vi "DAQ6363_SetCORestLevel.vi"(8 "error in (no error)":errorcluster caption="entrée d'erreur (pas d'erreur)", 10 "CO.Impulsion.ÉtatRepos":i32(ring)=10192 items=["Haut"=10192, "Bas"=10214], 11 "TaskIn":refnum<k21>) -> (0 "error out":errorcluster caption="sortie d'erreur", 3 "TaskOut":refnum<k21>)   [LabVIEW 2019]
uses:
  <resource>/objmgr/daqmx.rc
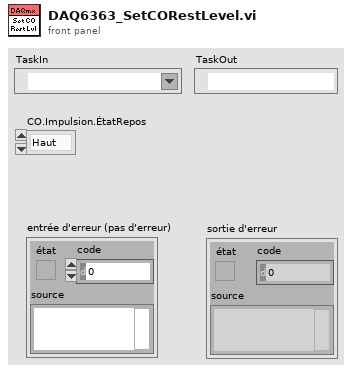
[diagram p1: front panel]
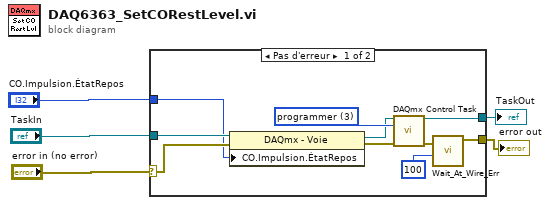
[diagram p0: block diagram]
diagram:
  n1 = case shown="Pas d'erreur" "error in (no error)" {
    selector: "error in (no error)" -> [w7 w16]
    tunnel: [w10 w16] -> w2
    tunnel: "TaskIn" -> [w9 w17]
    tunnel: [w8 w17] -> w3
    tunnel: "CO.Impulsion.ÉtatRepos" -> [w6 _]
    frame No Error {
      w15 = 3 items=["vérifier"=2, "réserver"=4, "programmer"=3, "libérer"=5, "abandonner"=6] ("action")
      n2 = property class="DAQmx - Voie"(reference=w9, error in=w7, "CO.Impulsion.ÉtatRepos"=w6) -> (reference out=w14:refnum<k21>, error out=w13:errorcluster)
      n3 = call <vilib>:"DAQmx Control Task.vi"("task/channels in"=w14, "action"=w15, "error in"=w13) -> ("task out"=w8:refnum<k21>, "error out"=w12:errorcluster)  [unwired: 11 in]
      n4 = call <userlib>:"Wait_At_Wire_Err.vi"("Wait (ms)"=u32 100, "error in (no error)"=w12) -> ("error out"=w10:errorcluster)  [unwired: 7 in, 2 out]
    }
    frame Error {
    }
  }
  "error out" <- w2
  "TaskOut" <- w3
